vi "ZCAN_ReadChannelStatus.vi"(1 "can_index_handle":u32, 3 "error in (no error)":errorcluster caption="错误输入（无错误）") -> (6 "ChannelStatus(string out)":string, 8 "error out":errorcluster caption="错误输出")   [LabVIEW 2011, in "zlgcan.lvlib"]
doc: "该函数用于读取 通道的状态信息。"
uses:
  zlgcan.lvlib
  data_type/ZCAN_CHANNEL_STATUS.ctl
  bin/ControlCANFD.dll
panel:
  in  "ZCAN_CHANNEL_STATUS":T1
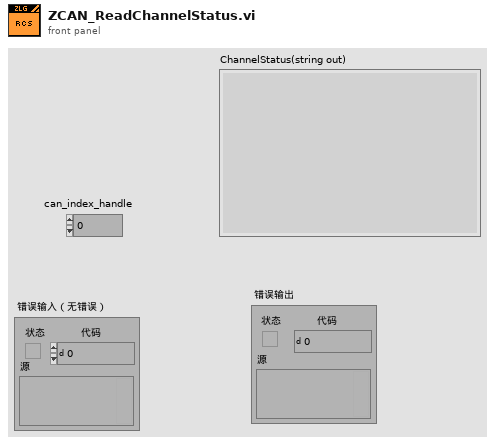
[diagram p1: front panel]
types:
  T1 = typedef "ZCAN_CHANNEL_STATUS.ctl" = cluster{"errInterrupt":u8, "regMode":u8, "regStatus":u8, "regALCapture":u8, "regECCapture":u8, "regEWLimit":u8, "regRECounter":u8, "regTECounter":u8, "Reserved":u32}
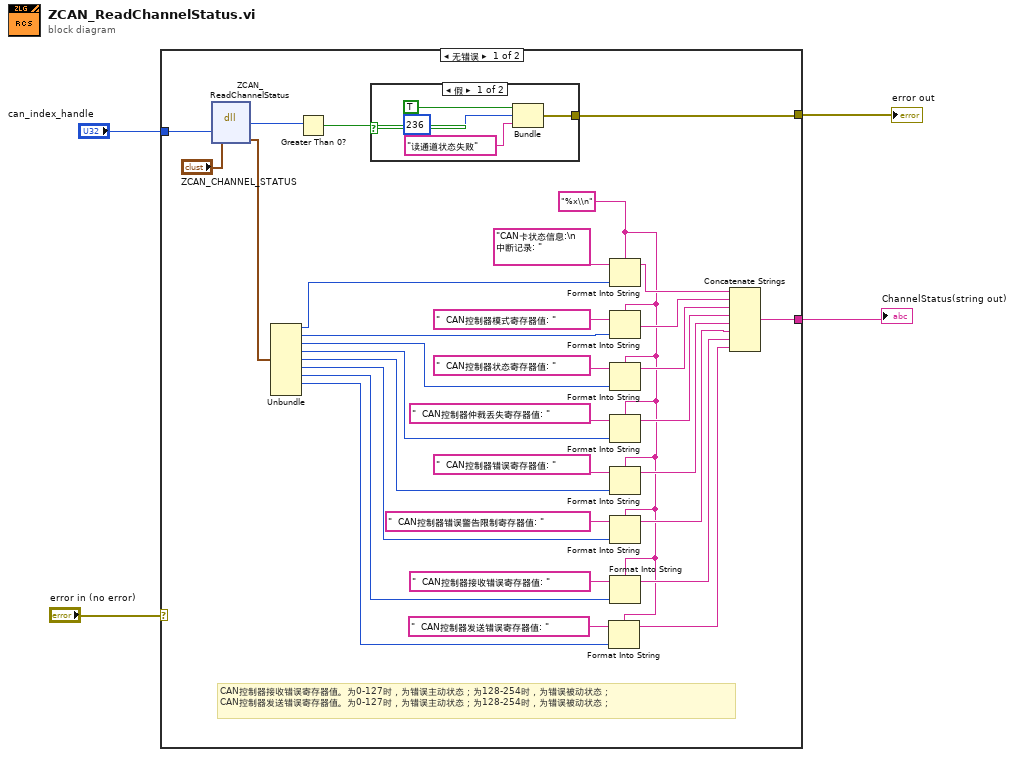
[diagram p0: block diagram]
diagram:
  n1 = case shown="无错误" "error in (no error)" {
    selector: "error in (no error)" -> [_ w41]
    tunnel: [w33 w41] -> w2
    tunnel: "can_index_handle" -> [w36 _]
    tunnel: [w5 _] -> w1
    frame No Error {
      w6 = "%x\\n" ("format string")
      # "CAN控制器接收错误寄存器值。为0-127时，为错误主动状态；为128-254时，为错误被动状态；\nCAN控制器发送错误寄存器值。为0-127时，为错误主动状态；为128-254时，为错误被动状态；"
      n2 = dll-call lib="C:/Users/ttc52/Desktop/DHC FD LV2018/LABIVIEW2011 CANFD Tool_V1.2.4_x86_20250428/bin/ControlCANFD.dll" fn="ZCAN_ReadChannelStatus"("channel_handle"=w36, "pCANStatus"="ZCAN_CHANNEL_STATUS") -> ("return"=w35:u32, "pCANStatus"=w31:T1)  [unwired: 4 in, 2 out]
      n3 = Unbundle(w31) -> ("errInterrupt"=w18:u8, "regMode"=w17:u8, "regStatus"=w16:u8, "regALCapture"=w15:u8, "regECCapture"=w14:u8, "regEWLimit"=w11:u8, "regRECounter"=w10:u8, "regTECounter"=w9:u8)  [unwired: 1 out]
      n4 = Greater Than 0?(x=w35) -> (x > 0?=w34:bool)
      n5 = case shown="假" w34 {
        tunnel: [w37 _] -> w33
        frame False {
          n6 = Bundle("status"=TRUE, "code"=236, "消息"="读通道状态失败") -> (w37:cluster{"status":bool, "code":i32, "消息":string})  [unwired: 1 in]
        }
        frame True {
        }
      }
      n7 = Format Into String(format string=w6, initial string="  CAN控制器发送错误寄存器值: ", w9) -> (resulting string=w7:string)  [unwired: 1 in, 1 out]
      n8 = Format Into String(format string=w6, initial string="CAN卡状态信息:\n  中断记录: ", w18) -> (resulting string=w28:string)  [unwired: 1 in, 1 out]
      n9 = Format Into String(format string=w6, initial string="  CAN控制器模式寄存器值: ", w17) -> (resulting string=w27:string)  [unwired: 1 in, 1 out]
      n10 = Format Into String(format string=w6, initial string="  CAN控制器状态寄存器值: ", w16) -> (resulting string=w30:string)  [unwired: 1 in, 1 out]
      n11 = Format Into String(format string=w6, initial string="  CAN控制器仲裁丢失寄存器值: ", w15) -> (resulting string=w22:string)  [unwired: 1 in, 1 out]
      n12 = Format Into String(format string=w6, initial string="  CAN控制器错误寄存器值: ", w14) -> (resulting string=w21:string)  [unwired: 1 in, 1 out]
      n13 = Format Into String(format string=w6, initial string="  CAN控制器错误警告限制寄存器值: ", w11) -> (resulting string=w20:string)  [unwired: 1 in, 1 out]
      n14 = Format Into String(format string=w6, initial string="  CAN控制器接收错误寄存器值: ", w10) -> (resulting string=w8:string)  [unwired: 1 in, 1 out]
      n15 = Concatenate Strings(w28, w27, w30, w22, w21, w20, w8, w7) -> (w5:string)
    }
    frame Error {
    }
  }
  "error out" <- w2
  "ChannelStatus(string out)" <- w1
